vi "Tortoisegitproc default path.vi"() -> (2 "file or folder exists?":bool, 3 "TortoiseGitProc.exe":path)   [LabVIEW 2017]
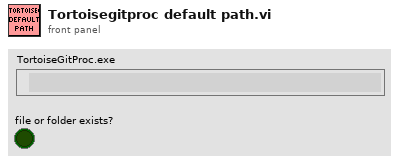
[diagram p1: front panel]
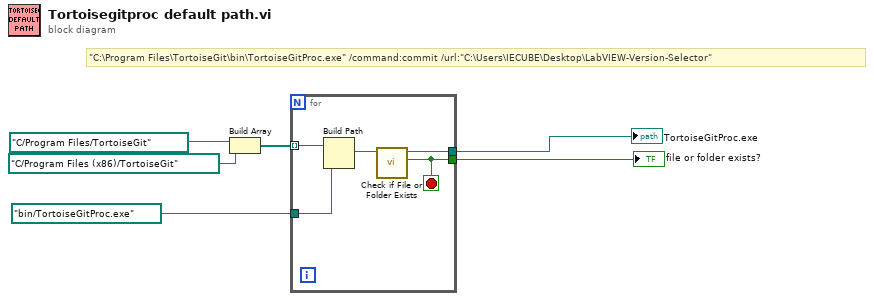
[diagram p0: block diagram]
diagram:
  # "\"C:\\Program Files\\TortoiseGit\\bin\\TortoiseGitProc.exe\" /command:commit /url:\"C:\\Users\\IECUBE\\Desktop\\LabVIEW-Version-Selector\""
  n1 = Build Array(path "C:/Program Files/TortoiseGit", path "C:/Program Files (x86)/TortoiseGit") -> (w4:path[])
  n2 = for {
    tunnel: w4 -> [w11] mode=indexing
    tunnel: path "bin/TortoiseGitProc.exe" -> [w10]
    tunnel: [w8] -> w1
    tunnel: [w7] -> w2
    stop <- w7 stop-if-true
    n3 = Build Path(base path=w11, name or relative path=w10) -> (appended path=w9:path)
    n4 = call <vilib>:"Check if File or Folder Exists.vi"("path"=w9) -> ("file or folder exists?"=w7:bool, "dup path"=w8:path)  [unwired: 8 in, 1 out]
  }
  "file or folder exists?" <- w2
  "TortoiseGitProc.exe" <- w1
